vi "Формула пористости.vi"(0 "Объем образца":dbl, 1 "V пористости P2/P1":dbl) -> (2 "Пористость %":dbl, 3 "объем скелета":dbl, 4 "Y":dbl)   [LabVIEW 2018]
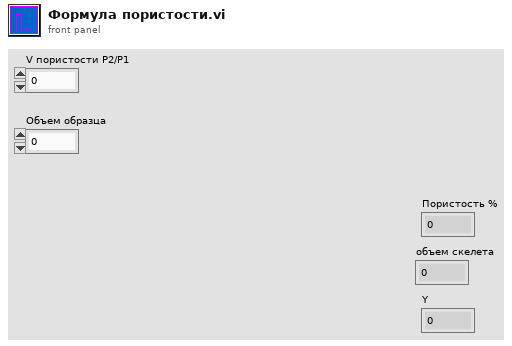
[diagram p1: front panel]
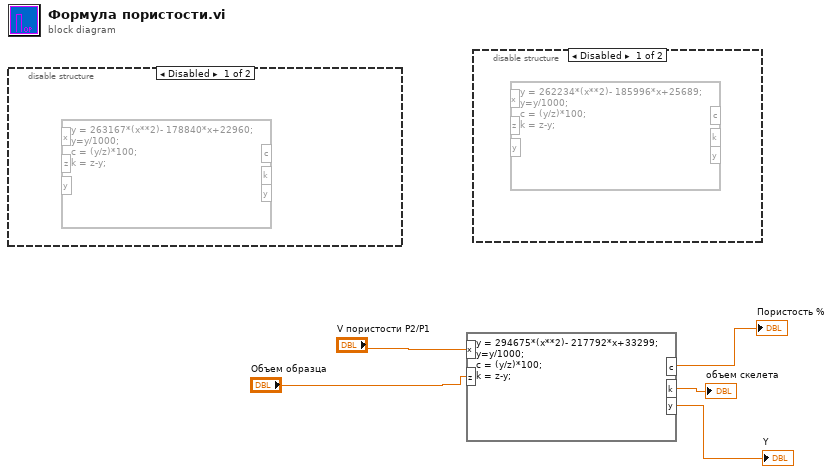
[diagram p0: block diagram]
diagram:
  n1 = disable-structure shown="Disabled" {
    frame Disabled {
      n2 = formula code="y = 263167*(x**2)- 178840*x+22960;\ny=y/1000;\nc = (y/z)*100;\nk = z-y;"() -> ()  [unwired: 3 in, 3 out]
    }
    frame Enabled {
    }
  }
  n3 = formula code="y = 294675*(x**2)- 217792*x+33299;\ny=y/1000;\nc = (y/z)*100;\nk = z-y;"("x"="V пористости P2/P1", "z"="Объем образца") -> ("c"=→"Пористость %":dbl, "y"=→"Y":dbl, "k"=→"объем скелета":dbl)
  n4 = disable-structure shown="Disabled" {
    frame Disabled {
      n5 = formula code="y = 262234*(x**2)- 185996*x+25689;\ny=y/1000;\nc = (y/z)*100;\nk = z-y;"() -> ()  [unwired: 3 in, 3 out]
    }
    frame Enabled {
    }
  }
